vi "Vision Server Add Vision Update.vi"(1 "Targets Update":T2={"Valid?"=FALSE, "CapturedAtTimestamp"=0.0, "Targets Message"={"capturedAgoMs"=0, "targets"=[{"x"=0.0, "y"=0.0, "z"=0.0, "theta"=0.0}]}}, 2 "Vision Server":T1={"connection ID"=refnum, "Running?"=TRUE, "TCP Port"=65535, "LastMessageReceivedTime"=0.0, "WantsAppRestart"=FALSE, "IsConnect"=FALSE, "Targets Updates"=[{"Valid?"=FALSE, "CapturedAtTimestamp"=0.0, "Targets Message"={"capturedAgoMs"=0, "targets"=[{"x"=0.0, "y"=0.0, "z"=0.0, "theta"=0.0}]}}]}) -> (0 "Vision Server":T1={"connection ID"=refnum, "Running?"=TRUE, "TCP Port"=65535, "LastMessageReceivedTime"=0.0, "WantsAppRestart"=FALSE, "IsConnect"=FALSE, "Targets Updates"=[{"Valid?"=FALSE, "CapturedAtTimestamp"=0.0, "Targets Message"={"capturedAgoMs"=0, "targets"=[{"x"=0.0, "y"=0.0, "z"=0.0, "theta"=0.0}]}}]})   [LabVIEW 2016]
uses:
  Vision Server.ctl
  Messages/Targets/Targets Update.ctl
  Messages/Targets/Targets Message.ctl
  Messages/Targets/Targets Info.ctl
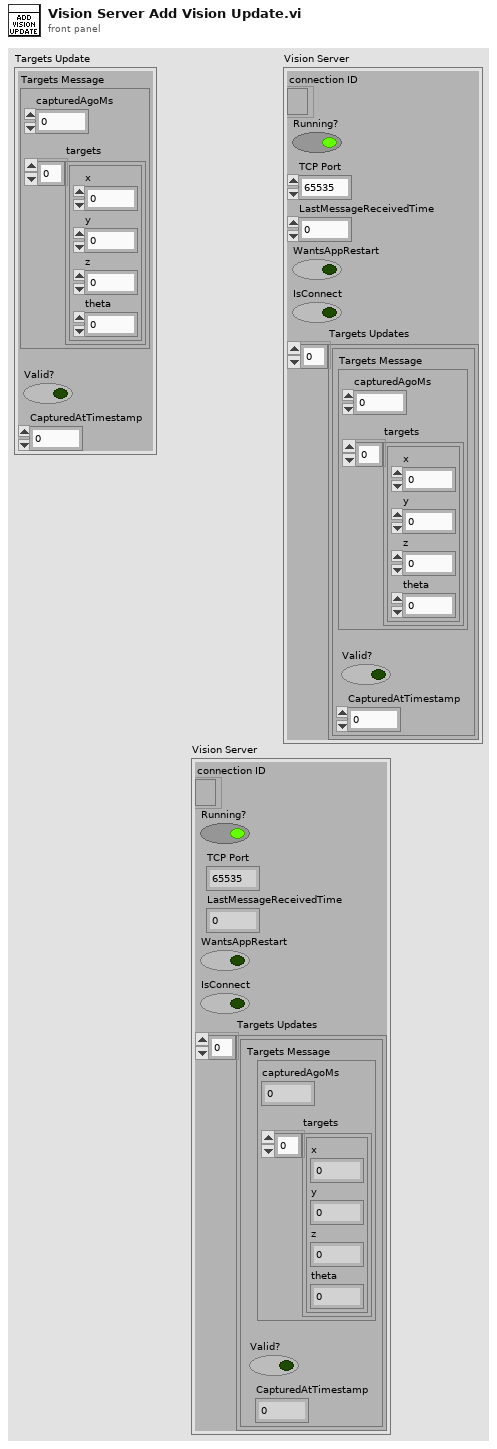
[diagram p1: front panel]
types:
  T1 = typedef "Vision Server.ctl" = cluster{"connection ID":refnum<k5>, "Running?":bool, "TCP Port":u16, "LastMessageReceivedTime":dbl, "WantsAppRestart":bool, "IsConnect":bool, "Targets Updates":T2[]}
  T2 = typedef "Targets Update.ctl" = cluster{"Valid?":bool, "CapturedAtTimestamp":dbl, "Targets Message":T3}
  T3 = typedef "Targets Message.ctl" = cluster{"capturedAgoMs":i32, "targets":T4[]}
  T4 = typedef "Targets Info.ctl" = cluster{"x":dbl, "y":dbl, "z":dbl, "theta":dbl}
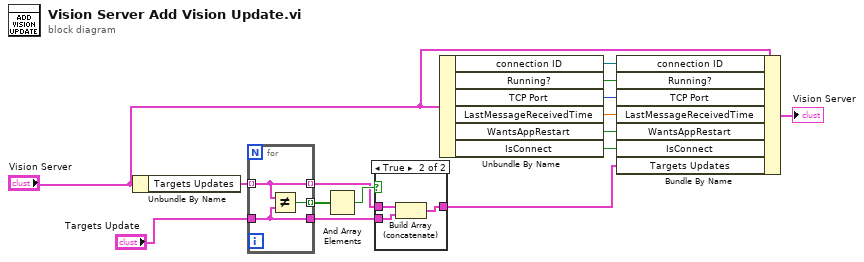
[diagram p0: block diagram]
diagram:
  n1 = Unbundle By Name("Vision Server") -> ("Targets Updates"=w15:T2[])
  n2 = for {
    tunnel: w15 -> [w17] mode=indexing
    tunnel: "Targets Update" -> [w16]
    tunnel: [w18] -> w14 mode=indexing
    tunnel: [w17] -> w12 mode=indexing
    tunnel: [w16] -> w11
    n3 = Not Equal?(x=w17, y=w16) -> (x != y?=w18:bool)
  }
  n4 = And Array Elements(Boolean array=w14) -> (logical AND=w13:bool)
  n5 = case shown="True" w13 {
    tunnel: w12 -> [w19 w22]
    tunnel: w11 -> [_ w21]
    tunnel: [w19 w20] -> w4
    frame False {
    }
    frame True {
      n6 = Build Array (concatenate)(w22, w21) -> (w20:T2[])
    }
  }
  n7 = Unbundle By Name("Vision Server") -> ("connection ID"=w10:refnum<k5>, "Running?"=w9:bool, "TCP Port"=w8:u16, "LastMessageReceivedTime"=w7:dbl, "WantsAppRestart"=w6:bool, "IsConnect"=w5:bool)
  n8 = Bundle By Name(cluster="Vision Server", "connection ID"=w10, "Running?"=w9, "TCP Port"=w8, "LastMessageReceivedTime"=w7, "WantsAppRestart"=w6, "IsConnect"=w5, "Targets Updates"=w4) -> (→"Vision Server":T1)
